vi "ReadMovie.vi"() -> ()   [LabVIEW 2015]
uses:
  <vilib>/UPVI/lvhdf5/library.llb/HDF5 Ref.ctl
  <vilib>/UPVI/lvhdf5/attribute.llb/Read Multiple Attributes (Variant).vi
  <vilib>/Utility/VariantDataType/GetClusterInfo.vi
  <vilib>/Utility/VariantDataType/VariantType.lvlib
  <vilib>/Utility/VariantDataType/GetTypeInfo.vi
  <vilib>/UPVI/lvhdf5/attribute.llb/Attribute Array to Cluster.xnode
  <vilib>/UPVI/lvhdf5/attribute.llb/LVH5 Read Attributes.xnode
  <vilib>/UPVI/lvhdf5/group.llb/H5G_obj_t.ctl
panel:
  out "Obect Types":T1[](array[typedef]) items=["H5G_UNKNOWN"=-1, "H5G_GROUP"=0, "H5G_DATASET"=1, "H5G_TYPE"=2, "H5G_LINK"=3, "H5G_UDLINK"=4]
  out "Object Names":string[](array[string])
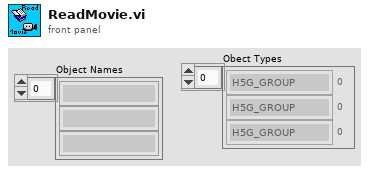
[diagram p1: front panel]
types:
  T1 = typedef "H5G_obj_t.ctl" = i32
  T2 = typedef "HDF5 Ref.ctl" = refnum<k1>
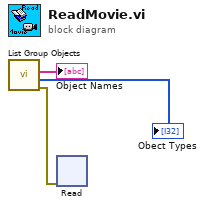
[diagram p0: block diagram]
diagram:
  n1 = call <vilib>:"List Group Objects.vi"() -> ("error out"=w2:errorcluster, "Obect Types"=→"Obect Types":T1[], "Object Names"=→"Object Names":string[], "HDF5 Loc Ref out"=w3:T2)  [unwired: 6 in]
  n2 = xnode "Read"("error in (no error)"=w2) -> ("error out"=w1:errorcluster)  [unwired: 3 in, 3 out]
